vi "HTTPMethod_getHelloClassique.vi"(7 "LabVIEW Web Service Request":refnum<class "Web Request.lvclass">) -> ()   [LabVIEW 2020]
uses:
  <vilib>/wsapi/Web Request.lvclass
panel:
  out "error out":errorcluster
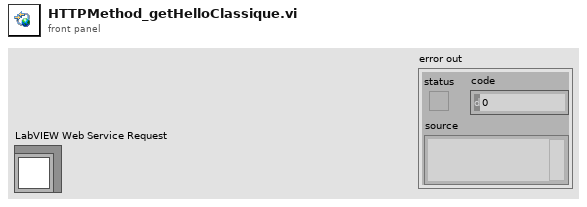
[diagram p1: front panel]
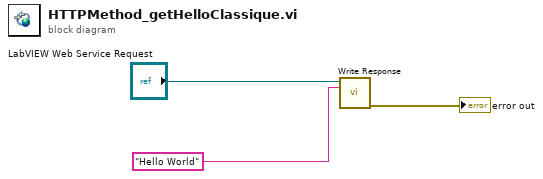
[diagram p0: block diagram]
diagram:
  n1 = call <vilib>:"Write Response.vi"("LabVIEW Web Service Request"="LabVIEW Web Service Request", "response string"="Hello World") -> ("error out"=→"error out":errorcluster)  [unwired: 12 in, 1 out]
